vi "FindMessageStart.vi"(8 "error in (no error)":errorcluster, 11 "TCP_Server_Connection_Handler in":refnum<class "TCP_Server_Connection_Handler.lvclass">) -> (0 "error out":errorcluster, 3 "TCP_Server_Connection_Handler out":refnum<class "TCP_Server_Connection_Handler.lvclass">)   [LabVIEW 2023, in "TCP_Server_Connection_Handler.lvlib" / "TCP_Server_Connection_Handler.lvclass"]
uses:
  TCP_Server_Connection_Handler.lvclass
  <vilib>/ActorFramework/Actor/Actor.lvclass/Actor.ctl
  <vilib>/ActorFramework/Message Enqueuer/Message Enqueuer.lvclass/Message Enqueuer.ctl
  TCP_Server_Connection_Handler.lvclass/TCP_Server_Connection_Handler.ctl
  <vilib>/ActorFramework/Message Enqueuer/Init from Existing Queue.vi
  <vilib>/ActorFramework/Message Enqueuer/Enqueue.vi
  TCP_Server_Connection_Handler Messages/FindMessageStart Msg/FindMessageStart Msg.lvclass
  TCP_Server_Connection_Handler Messages/GetMessageLength Msg/GetMessageLength Msg.lvclass
  <vilib>/ActorFramework/Stop Msg/Stop Msg.lvclass
  <vilib>/ActorFramework/Message Priority Queue/Priority Enqueue.vi
  <vilib>/ActorFramework/Message Enqueuer/Message Enqueuer.lvclass
  <vilib>/ActorFramework/Actor/Actor.lvclass
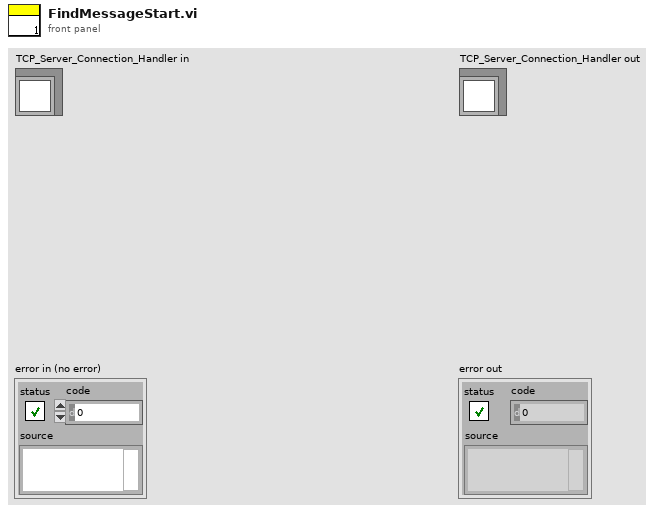
[diagram p1: front panel]
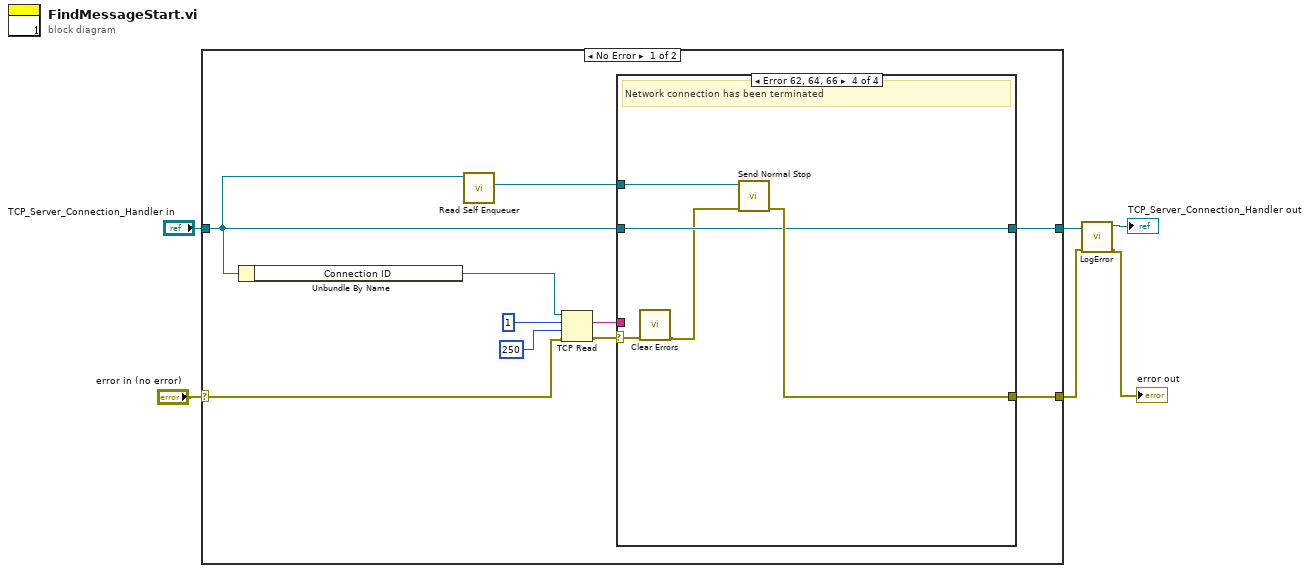
[diagram p0: block diagram]
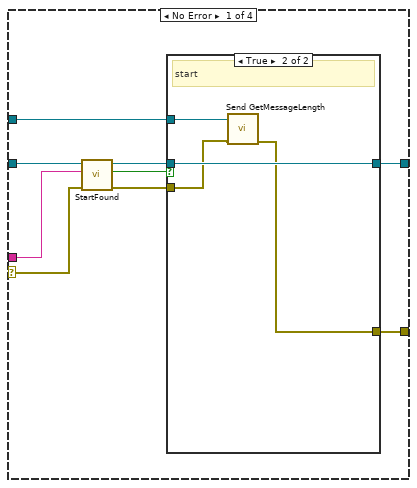
[diagram p2: hidden frame]
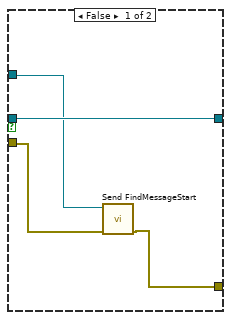
[diagram p3: hidden frame]
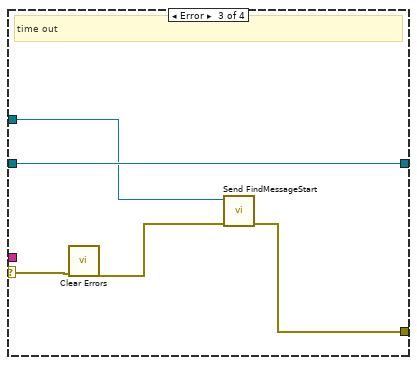
[diagram p5: hidden frame]
diagram:
  n1 = case shown="No Error" "error in (no error)" {
    selector: "error in (no error)" -> [w10 w47]
    tunnel: [w9 w47] -> w2
    tunnel: [w11 w46] -> w4
    tunnel: "TCP_Server_Connection_Handler in" -> [w8 w46]
    frame No Error {
      n2 = Unbundle By Name(w8) -> ("Connection ID"=w16:refnum<k5>)
      n3 = call <vilib>:"Read Self Enqueuer.vi"("Actor"=w8) -> ("Self Enqueuer"=w7:refnum<class "Message Enqueuer.lvclass">)  [unwired: 10 in]
      n4 = TCP Read(connection ID=w16, bytes to read=1, error in (no error)=w10, 9:250 ("timeout ms (25000)")) -> (data out=w12:string, error out=w13:errorcluster)  [unwired: 1 in, 1 out]
      n5 = case shown="Error 62, 64, 66" w13 {
        selector: w13 -> [w23 w34 w39 w42]
        tunnel: w8 -> [w25 w35 w40 w43]
        tunnel: w12 -> [w24 _ _ _]
        tunnel: [w19 w35 w40 w43] -> w11
        tunnel: [w18 w34 w37 w44] -> w9
        tunnel: w7 -> [w17 _ w38 w45]
        frame No Error {
          n6 = call "StartFound.vi"("error in (no error)"=w23, "String"=w24, "TCP_Server_Connection_Handler in"=w25) -> ("error out"=w20:errorcluster, "Start?"=w22:bool, "TCP_Server_Connection_Handler out"=w21:refnum<class "TCP_Server_Connection_Handler.lvclass">)  [unwired: 6 in]
          n7 = case shown="True" w22 {
            tunnel: w21 -> [w29 w33]
            tunnel: w20 -> [w27 w31]
            tunnel: [w29 w33] -> w19
            tunnel: [w26 w30] -> w18
            tunnel: w17 -> [w28 w32]
            frame False {
              n8 = call "Send FindMessageStart.vi"("error in (no error)"=w27, "Message Enqueuer"=w28) -> ("error out"=w26:errorcluster)  [unwired: 8 in, 1 out]
            }
            frame True {
              # "start"
              n9 = call "Send GetMessageLength.vi"("error in (no error)"=w31, "Message Enqueuer"=w32) -> ("error out"=w30:errorcluster)  [unwired: 8 in, 1 out]
            }
          }
        }
        frame Default {
        }
        frame Error {
          # "time out"
          n10 = call <vilib>:"Clear Errors.vi"("error in (no error)"=w39) -> ("error out"=w36:errorcluster)  [unwired: 5 in, 1 out]
          n11 = call "Send FindMessageStart.vi"("error in (no error)"=w36, "Message Enqueuer"=w38) -> ("error out"=w37:errorcluster)  [unwired: 8 in, 1 out]
        }
        frame Error {
          # "Network connection has been terminated"
          n12 = call <vilib>:"Clear Errors.vi"("error in (no error)"=w42) -> ("error out"=w41:errorcluster)  [unwired: 5 in, 1 out]
          n13 = call <vilib>:"Send Normal Stop.vi"("error in (no error)"=w41, "Message Enqueuer"=w45) -> ("error out"=w44:errorcluster)  [unwired: 9 in]
        }
      }
    }
    frame Error {
    }
  }
  n14 = call "LogError.vi"("error in (no error)"=w2, "TCP_Server_Connection_Handler in"=w4) -> ("error out"=→"error out":errorcluster, "TCP_Server_Connection_Handler out"=→"TCP_Server_Connection_Handler out":refnum<class "TCP_Server_Connection_Handler.lvclass">)  [unwired: 8 in]
